vi "Test FFT1.vi"(0 "Buffer in":u16[](array[numeric]), 1 "FFT parameters":T1={"window"=1, "view"={"dB On (F)"=FALSE, "unwrap phase (F)"=FALSE, "convert to degree (F)"=FALSE}, "#A-lines"=2048, "start pixel"=0, "#pixels to save"=300} {"window" items=["Rectangle"=0, "Hanning"=1, "Hamming"=2, "Blackman-Harris"=3, "Exact Blackman"=4, "Blackman"=5, "Flat Top"=6, "4 Term B-Harris "=7, "7 Term B-Harris"=8, "Low Sidelobe"=9, "Blackman Nuttall"=11, "Triangle"=30, "Bartlett-Hanning"=31, "Bohman"=32, "Parzen"=33, "Welch"=34, "Kaiser"=60, "Dolph-Chebyshev"=61, "Gaussian"=62]}, 11 "error in":errorcluster) -> (2 "Mag for display":sgl[][](array[numeric]), 3 "Phase for display":sgl[][](array[numeric]), 4 "Array":sgl[][](array[numeric]), 6 "Array 2":sgl[][](array[numeric]), 15 "error out":errorcluster)   [LabVIEW 2018]
uses:
  General/type defines/FFT parameters.ctl
  <vilib>/Analysis/4window.llb/windowTd.ctl
  <vilib>/measure/maspectr.llb/FFT Spectrum (Mag-Phase) for 1 Chan.vi
  <vilib>/measure/NI_MAPro.lvlib
  <vilib>/Analysis/NI_AALPro.lvlib
panel:
  in  "A*Log":i32
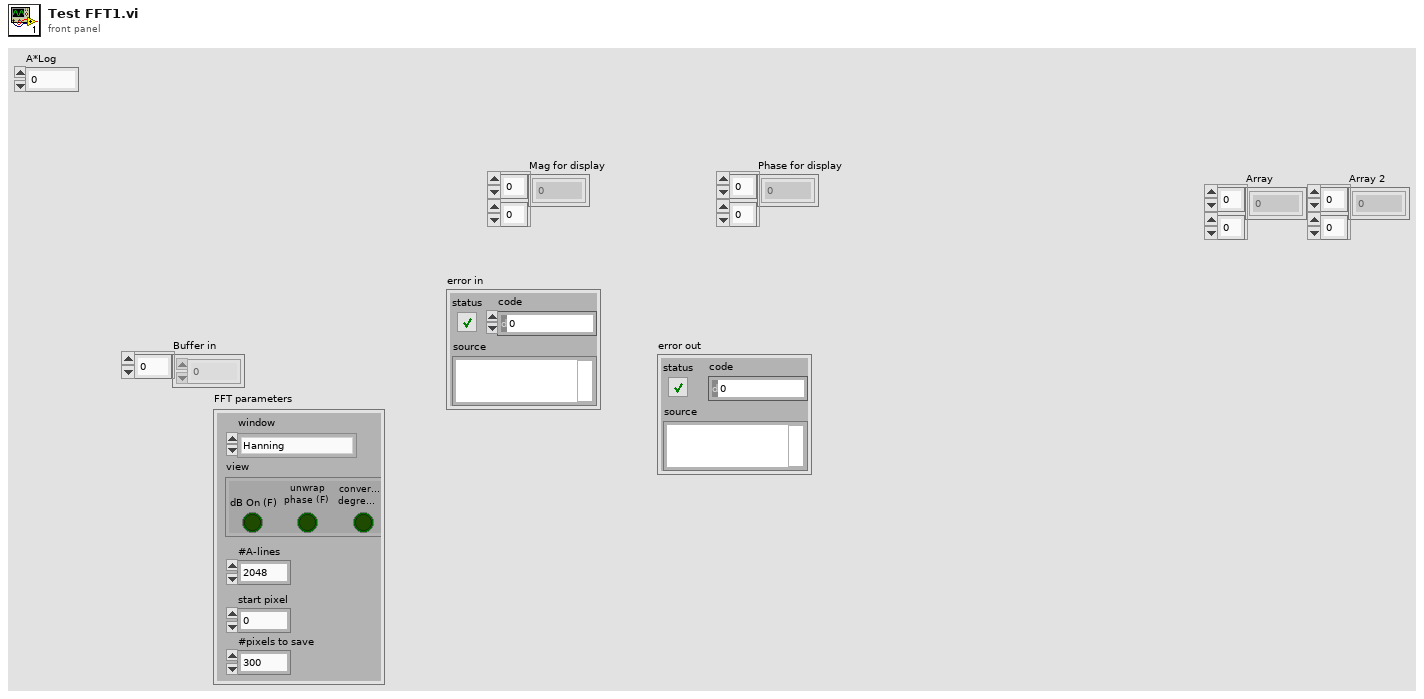
[diagram p1: front panel]
types:
  T1 = typedef "FFT parameters.ctl" = cluster{"window":T2, "view":cluster{"dB On (F)":bool, "unwrap phase (F)":bool, "convert to degree (F)":bool}, "#A-lines":i32, "start pixel":i32, "#pixels to save":i32}
  T2 = typedef "NI_AALPro.lvlib/windowTd.ctl" = u32
  T3 = cluster{"dB On (F)":bool, "unwrap phase (F)":bool, "convert to degree (F)":bool}
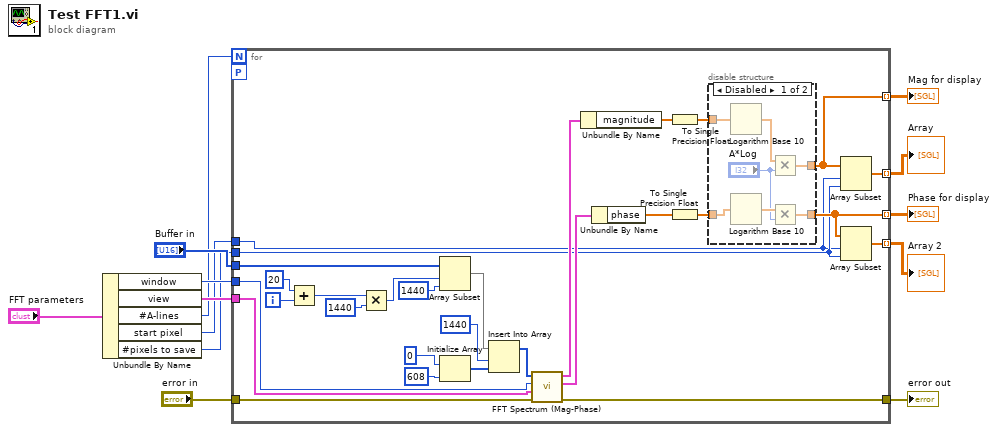
[diagram p0: block diagram]
diagram:
  n1 = Unbundle By Name("FFT parameters") -> ("window"=w10:T2, "view"=w9:T3, "#A-lines"=w3:i32, "start pixel"=w8:i32, "#pixels to save"=w7:i32)
  n2 = for {
    N: w3 -> [_]
    tunnel: "Buffer in" -> [w27]
    tunnel: "error in" -> [w17]
    workers-P: _ -> [_]
    tunnel: [w37] -> w2 mode=indexing
    tunnel: [w36] -> w1 mode=indexing
    tunnel: w7 -> [w15]
    tunnel: w8 -> [w14]
    tunnel: [w16] -> w11
    tunnel: w10 -> [w33]
    tunnel: w9 -> [w32]
    tunnel: [w20] -> w5 mode=indexing
    tunnel: [w19] -> w4 mode=indexing
    i -> [w25]
    n3 = Add(x=20, y=w25) -> (x+y=w23:i32)
    n4 = Multiply(x=w23, y=1440) -> (x*y=w41:i32)
    n5 = Array Subset(array=w27, index=w41, length=1440) -> (w22:u16[])
    n6 = Initialize Array(u16 0 ("element"), 608 ("dimension size")) -> (w29:u16[])
    n7 = Insert Into Array(array=w22, index=1440, new element=w29) -> (w26:u16[])
    n8 = call-poly <vilib>:"FFT Spectrum (Mag-Phase).vi"("error in (no error)"=w17, "view"=w32, "window"=w33, "time signal"=w26) -> ("error out"=w16:errorcluster, "phase"=w38:cluster{"f0":dbl, "df":dbl, "phase":dbl[]}, "magnitude"=w39:cluster{"f0":dbl, "df":dbl, "magnitude":dbl[]})  [unwired: 3 in, 2 out]
    n9 = Unbundle By Name(w39) -> ("magnitude"=w35:dbl[])
    n10 = Unbundle By Name(w38) -> ("phase"=w34:dbl[])
    n11 = To Single Precision Float(number=w35) -> (single precision float=w21:sgl[])
    n12 = To Single Precision Float(number=w34) -> (single precision float=w18:sgl[])
    n13 = disable-structure shown="Disabled" {
      disable-tunnel: w21 -> [w49 w51]
      disable-tunnel: [w45 w51] -> w20
      disable-tunnel: [w44 w50] -> w19
      disable-tunnel: w18 -> [w48 w50]
      frame Disabled {
        n14 = Logarithm Base 10(1:w49) -> (0:w47:sgl[])
        n15 = Logarithm Base 10(1:w48) -> (0:w46:sgl[])
        n16 = Multiply(x=w47, y="A*Log") -> (x*y=w45:sgl[])
        n17 = Multiply(x=w46, y="A*Log") -> (x*y=w44:sgl[])
      }
      frame Enabled {
      }
    }
    n18 = Array Subset(array=w20, index=w14, length=w15) -> (w37:sgl[])
    n19 = Array Subset(array=w19, index=w14, length=w15) -> (w36:sgl[])
  }
  "error out" <- w11
  "Mag for display" <- w5
  "Phase for display" <- w4
  "Array" <- w2
  "Array 2" <- w1
